vi "Test Component A Does Yet Another Thing.vi"(11 "Test Case In":refnum<class "Some Component A Test.lvclass">) -> (0 "error out":errorcluster, 3 "Test Case Out":refnum<class "Some Component A Test.lvclass">)   [LabVIEW 2020, in "Component A Test Suite.lvlib" / "Some Component A Test.lvclass"]
uses:
  Some Component A Test.lvclass
  C:/git/astemes-lunit/source/LUnit Test Case.lvclass
  Core/LUnit Test Case/LUnit Test Case.lvclass/LUnit Test Case.ctl
  6372d094-16df-45c0-a3b4-44e3e7ca520f.vi
  Core/LUnit Test Case/Private/Append Pass Result.vi
  Core/LUnit Test Case/Private/Append Fail Result.vi
  6372d094-16df-45c0-a3b4-44e3e7ca520f.vi/9c5d11cd-9439-4240-a1ee-d9baace9c924.vi
  Core/LUnit Test Case/Private/Run In UI.vi
  <vilib>/Utility/error.llb/Clear Errors.vi
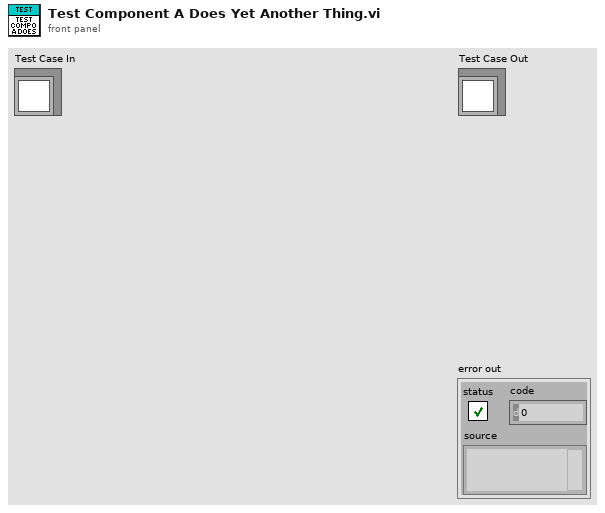
[diagram p1: front panel]
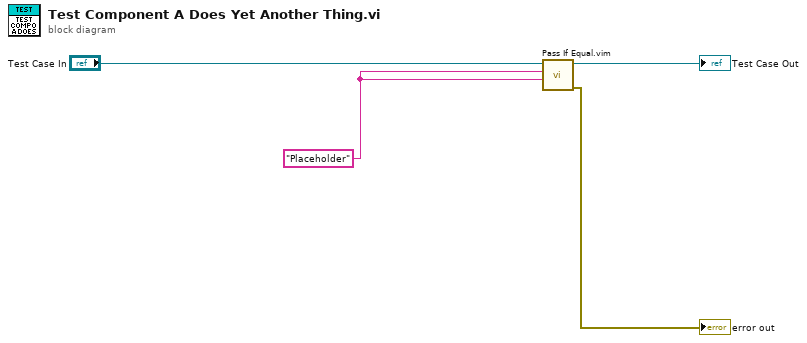
[diagram p0: block diagram]
diagram:
  w1 = "Placeholder"
  n1 = call "Pass If Equal.vim"("Actual"=w1, "Expected"=w1, "LUnit Test Case In"="Test Case In") -> ("error out"=→"error out":errorcluster, "LUnit Test Case Out"=→"Test Case Out":refnum<class "Some Component A Test.lvclass">)  [unwired: 7 in]
